vi "SFOAE-Compute Averages.vi"(0 "DataProc In":T1, 11 "error in (no error)":errorcluster) -> (4 "DataProc Out":T1, 8 "Graph Array":cluster{"Array":dbl[], "Array":dbl[]}[](array[cluster]), 15 "error out":errorcluster)   [LabVIEW 2020]
uses:
  Typedefs/SFOAE-Data Processing.ctl
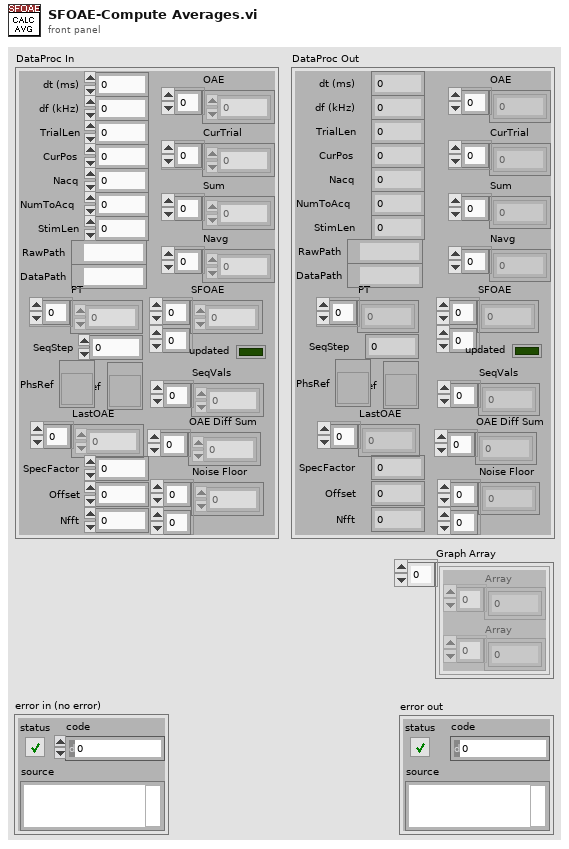
[diagram p1: front panel]
types:
  T1 = typedef "SFOAE-Data Processing.ctl" = cluster{"dt (ms)":dbl, "TrialLen":i32, "PT":cdb[], "CurPos":i32, "Sum":dbl[], "Navg":dbl[], "Nacq":i32, "RawPath":path, "DataPath":path, "NumToAcq":i32, "OAE":dbl[], "CurTrial":dbl[], "StimLen":i32, "SFOAE":cdb[][], "SeqStep":i32, "updated":bool, "SeqVals":dbl[], "df (kHz)":dbl, "MagRef":refnum<vi>, "LastOAE":dbl[], "OAE Diff Sum":dbl[], "Noise Floor":cdb[][], "SpecFactor":dbl, "Offset":i32, "Nfft":i32, "PhsRef":refnum<vi>}
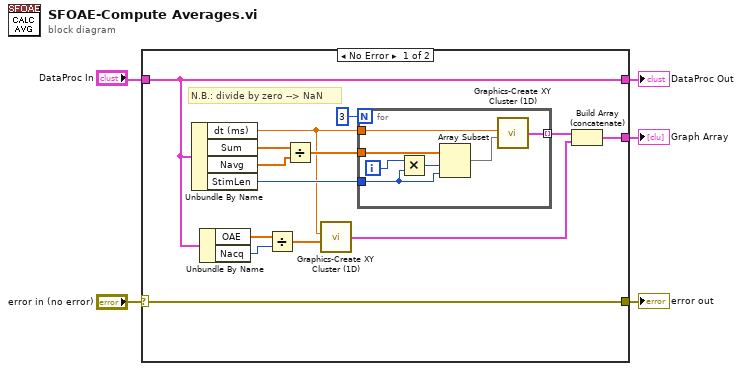
[diagram p0: block diagram]
diagram:
  n1 = case shown="No Error" "error in (no error)" {
    selector: "error in (no error)" -> [w19 w27]
    tunnel: "DataProc In" -> [w7 w28]
    tunnel: [w7 w28] -> w3
    tunnel: [w19 w27] -> w5
    tunnel: [w6 _] -> w1
    frame No Error {
      # "N.B.: divide by zero --> NaN"
      n2 = Unbundle By Name(w7) -> ("dt (ms)"=w8:dbl, "Sum"=w17:dbl[], "Navg"=w16:dbl[], "StimLen"=w14:i32)
      n3 = Unbundle By Name(w7) -> ("OAE"=w13:dbl[], "Nacq"=w12:i32)
      n4 = Divide(x=w13, y=w12) -> (x/y=w11:dbl[])
      n5 = Divide(x=w17, y=w16) -> (x/y=w15:dbl[])
      n6 = call "Graphics-Create XY Cluster (1D).vi"("Array"=w11, "dx"=w8) -> ("XY cluster"=w9:cluster{"Array":dbl[], "Array":dbl[]})  [unwired: 2 in]
      n7 = for {
        N: 3 -> [_]
        tunnel: w8 -> [w22]
        tunnel: w15 -> [w26]
        tunnel: w14 -> [w23]
        tunnel: [w20] -> w10 mode=indexing
        i -> [w24]
        n8 = Multiply(x=w24, y=w23) -> (x*y=w25:i32)
        n9 = Array Subset(array=w26, index=w25, length=w23) -> (w21:dbl[])
        n10 = call "Graphics-Create XY Cluster (1D).vi"("Array"=w21, "dx"=w22) -> ("XY cluster"=w20:cluster{"Array":dbl[], "Array":dbl[]})  [unwired: 2 in]
      }
      n11 = Build Array (concatenate)(w10, w9) -> (w6:cluster{"Array":dbl[], "Array":dbl[]}[])
    }
    frame Error {
    }
  }
  "error out" <- w5
  "DataProc Out" <- w3
  "Graph Array" <- w1
